vi "Get Generation Status.vi"(8 "error in (no error)":errorcluster) -> (0 "error out":errorcluster, 3 "generation status":T1)   [LabVIEW 2021, in "DigitalAudioGenerationProcess.lvlib"]
uses:
  DigitalAudioGenerationProcess.lvlib
  controls/generation status.ctl
  controls/AudioGenTypeDefs.lvlib
  <vilib>/addons/PointValueMap/PointValueMap.lvlib
  <vilib>/addons/PointValueMap/subVIs/Point_Read_variant.vi
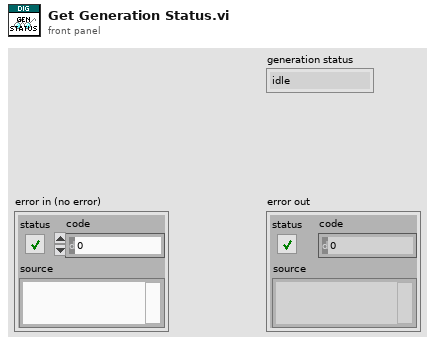
[diagram p1: front panel]
types:
  T1 = typedef "AudioGenTypeDefs.lvlib/generation status.ctl" = enum16{"idle", "committed", "generating"}
  T2 = typedef "PointValueMap.lvlib/PointMap.ctl" = refnum<data-value>
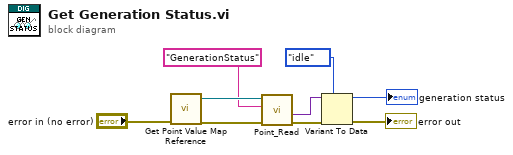
[diagram p0: block diagram]
diagram:
  n1 = call "Get Point Value Map Reference.vi"("error in (no error)"="error in (no error)") -> ("error out"=w8:errorcluster, "Map Out"=w7:T2)  [unwired: 9 in]
  n2 = call-poly <vilib>:"Point_Read.vi"("Error In"=w8, "Tag"="GenerationStatus", "Map"=w7) -> ("Error Out"=w5:errorcluster, "Value"=w4:variant)  [unwired: 3 in, 4 out]
  n3 = Variant To Data(error in=w5, type=generation_status."idle" ("status"), Variant=w4) -> (data=→"generation status":T1, error out=→"error out":errorcluster)
